vi "lia_host_chebyshev.vi"() -> ()   [LabVIEW 2009]
uses:
  <vilib>/rvi/interface/nirviOpenFPGA/nirviOpenFPGA.xnode
  FPGA Bitfiles/test_lia.lvproj_FPGA Target_lia_fpga_array.vi.lvbitx
  lia_fpga_array.vi
  <vilib>/FPGAPlugInAG/Pxi-7841r/nirviIntfOpen_PXI-7841R.vi
  <vilib>/rvi/interface/nirviMethod/nirviMethod.xnode
  <vilib>/Utility/error.llb/Merge Errors.vi
  <vilib>/LabVIEW Targets/FPGA/Rio/nirio_HostInterface/nirio_DMAStopAll.vi
  <vilib>/rvi/interface/common/niFpgaNodeNameForErrorReporting.ctl
  <vilib>/rvi/errors/niLvFpgaWhatHappensToTopLevelVI.ctl
  <vilib>/LabVIEW Targets/FPGA/Rio/nirio_HostInterface/nirio_DisableInterrupts.vi
  <vilib>/Utility/error.llb/Error Cluster From Error Code.vi
  <vilib>/rvi/errors/niLvFpgaAdjustHostInterfaceError.vi
  <vilib>/LabVIEW Targets/FPGA/Rio/nirio_HostInterface/nirio_Reset.vi
  <vilib>/RVI Host/nirviSupport.llb/nirviErrorClusterFromErrorCode.vi
  <vilib>/LabVIEW Targets/FPGA/Rio/nirio_HostInterface/nirio_EnableInterrupts.vi
  <vilib>/rvi/errors/niLvFpgaReportInternalErrorWithAdditionalInfo.vi
  <vilib>/rvi/interface/nirviReadWriteControl/nirviReadWriteControl.xnode
  <vilib>/LabVIEW Targets/FPGA/Rio/nirio_HostInterface/nirio_WriteBig.vi
  <vilib>/LabVIEW Targets/FPGA/Rio/nirio_HostInterface/nirio_ReadBig.vi
  <vilib>/rvi/interface/nirviCloseFPGA/nirviCloseFPGA.xnode
  <vilib>/FPGAPlugInAG/Pxi-7841r/nirviIntfClose_PXI-7841R.vi
  <vilib>/userDefined/High Color/nirio_resource_hc.ctl
  NiRioSrv.dll
panel:
  in  "Time Constant [s] 4":dbl caption="Time Constant [s]"
  out "Y [V] 4":dbl caption="Y [V]"
  out "Phase [Deg] 4":dbl caption="Phase [Deg]"
  out "R [V] 4":dbl caption="R [V]"
  out "X [V] 4":dbl
  in  "Filter Rolloff 4":enum8{"6 dB", "12 dB", "18 dB", "24 dB"}(ring) caption="Filter Rolloff"
  in  "Amplitude [V] 4":dbl caption="Amplitude [V]"
  in  "Frequency [Hz] 4":dbl caption="Frequency [Hz]"
  in  "Phase Shift [Deg] 4":dbl caption="Phase Shift [Deg]"
  in  "Time Constant [s] 3":dbl caption="Time Constant [s]"
  out "Y [V] 3":dbl caption="Y [V]"
  out "Phase [Deg] 3":dbl caption="Phase [Deg]"
  out "R [V] 3":dbl caption="R [V]"
  out "X [V] 3":dbl
  in  "Filter Rolloff 3":enum8{"6 dB", "12 dB", "18 dB", "24 dB"}(ring) caption="Filter Rolloff"
  in  "Amplitude [V] 3":dbl caption="Amplitude [V]"
  in  "Frequency [Hz] 3":dbl caption="Frequency [Hz]"
  in  "Phase Shift [Deg] 3":dbl caption="Phase Shift [Deg]"
  in  "Time Constant [s] 2":dbl caption="Time Constant [s]"
  out "Y [V] 2":dbl caption="Y [V]"
  out "Phase [Deg] 2":dbl caption="Phase [Deg]"
  out "R [V] 2":dbl caption="R [V]"
  out "X [V] 2":dbl
  in  "Filter Rolloff 2":enum8{"6 dB", "12 dB", "18 dB", "24 dB"}(ring) caption="Filter Rolloff"
  in  "Amplitude [V] 2":dbl caption="Amplitude [V]"
  in  "Frequency [Hz] 2":dbl caption="Frequency [Hz]"
  in  "Phase Shift [Deg] 2":dbl caption="Phase Shift [Deg]"
  in  "Time Constant [s]":dbl
  out "Y [V]":dbl
  out "Phase [Deg]":dbl
  out "R [V]":dbl
  out "X [V]":dbl
  in  "Data Rate [Hz]":dbl
  in  "Filter Rolloff":enum8{"6 dB", "12 dB", "18 dB", "24 dB"}(ring)
  in  "stop":bool
  in  "Update Freq [Hz]":dbl
  in  "Amplitude [V]":dbl
  in  "Frequency [Hz]":dbl
  in  "Phase Shift [Deg]":dbl
  # "Lockin Amplifier 1"
  # "Lockin Amplifier 3"
  # "Filter Settings"
  # "Output"
  # "Filter Settings"
  # "Output"
  # "Reference Signal Settings"
  # "Reference Signal Settings"
  # "Lockin Amplifier 2"
  # "Lockin Amplifier 4"
  # "Filter Settings"
  # "Output"
  # "Filter Settings"
  # "Output"
  # "Global"
  # "Reference Signal Settings"
  # "Reference Signal Settings"
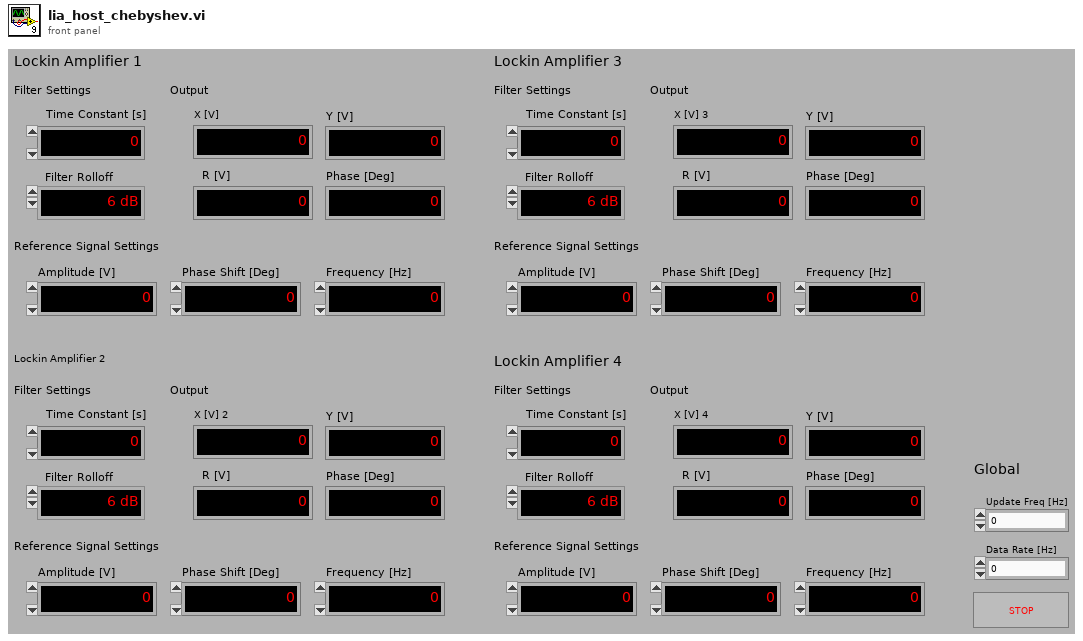
[diagram p1: front panel]
types:
  T1 = typedef "niFpgaNodeNameForErrorReporting.ctl" = enum16{"Open FPGA VI Reference", "Read/Write Control", "Invoke Method: Abort", "Invoke Method: Acknowledge IRQ", "Invoke Method: Download", "Invoke Method: FIFO.Configure", "Invoke Method: FIFO.Read", "Invoke Method: FIFO.Start", "Invoke Method: FIFO.Stop", "Invoke Method: FIFO.Write", "Invoke Method: Reset", "Invoke Method: Run", "Invoke Method: Wait on IRQ", "Close FPGA VI Reference"}
  T2 = typedef "niLvFpgaWhatHappensToTopLevelVI.ctl" = enum16{"top level VI scripted behind XNode", "top level VI inlined behind XNode"}
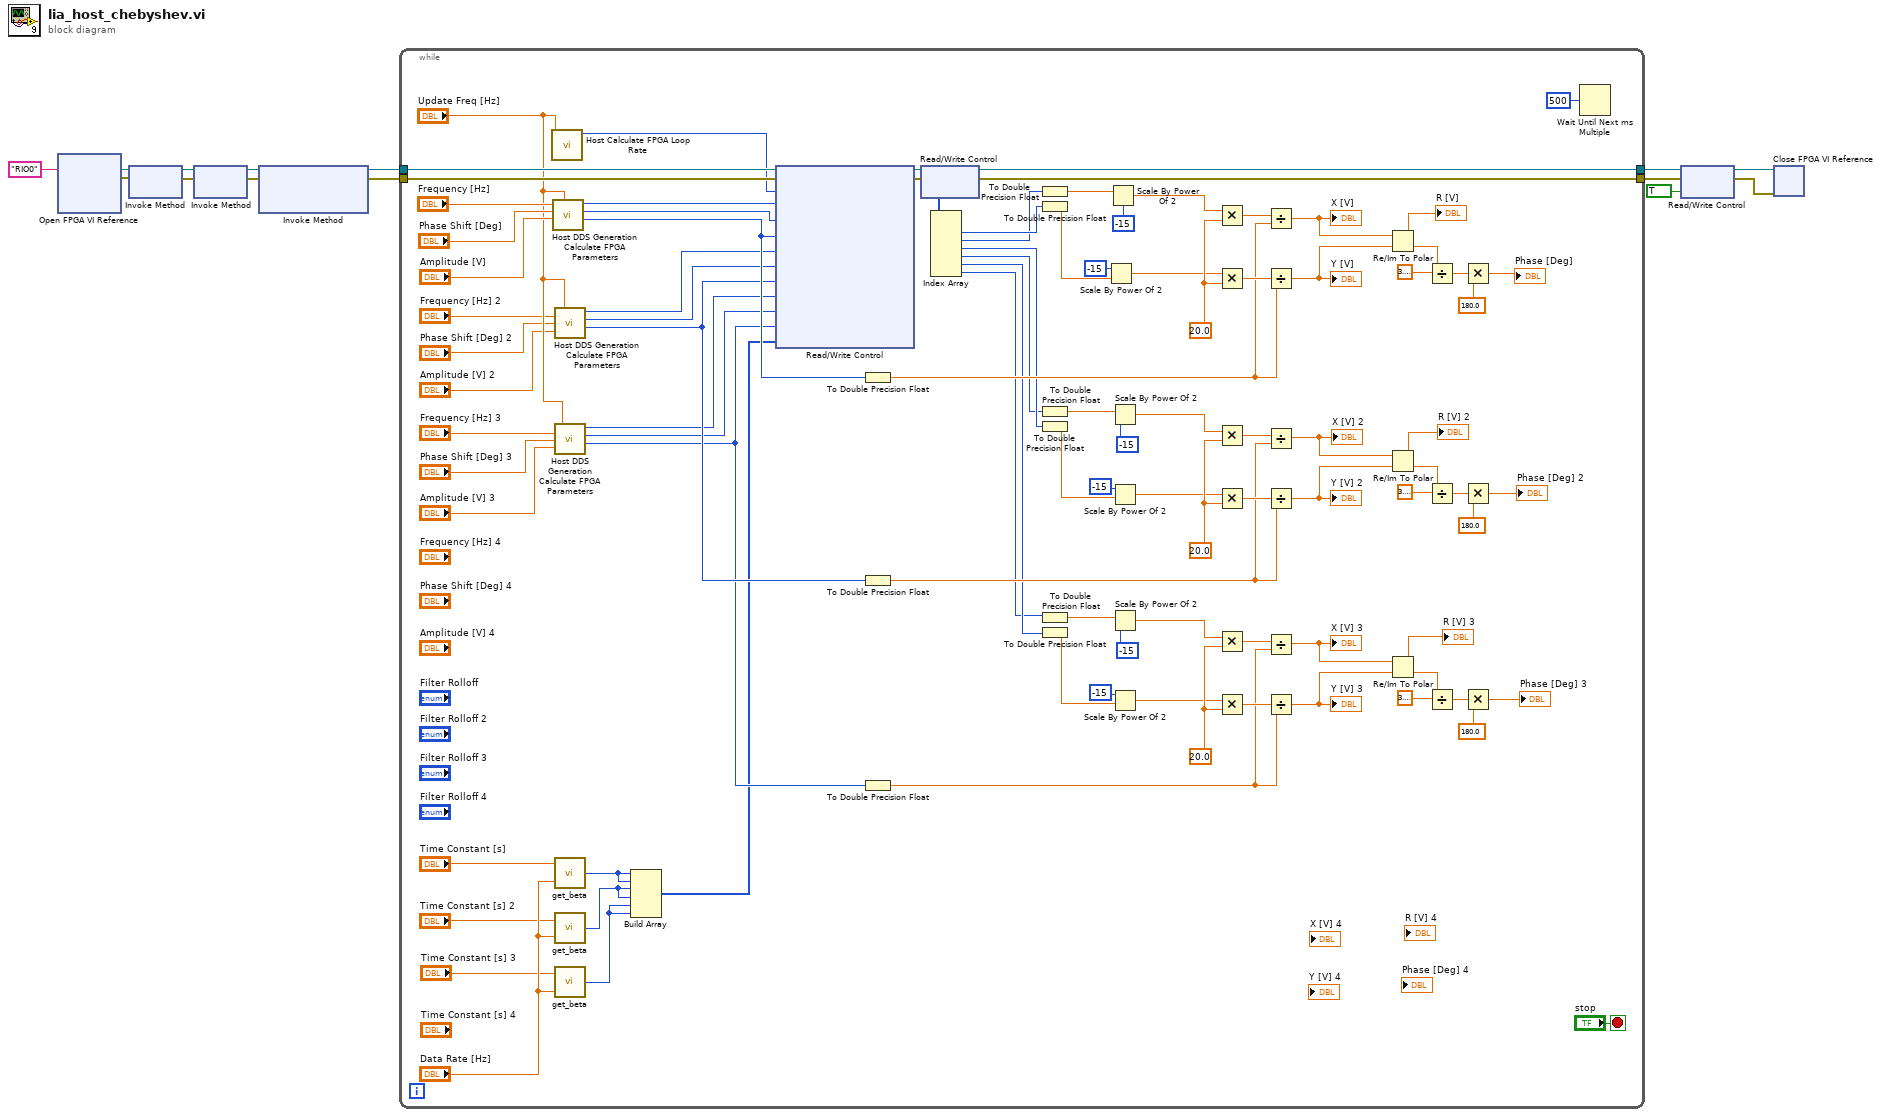
[diagram p0: block diagram]
diagram:
  n1 = xnode "Open FPGA VI Reference"("resource name"="RIO0") -> ("FPGA VI Reference Out"=w9:refnum<k20>, "error out"=w8:errorcluster)  [unwired: 1 in]
  n2 = xnode "Invoke Method"("FPGA VI Reference In"=w9, "error in"=w8) -> ("FPGA VI Reference Out"=w13:refnum<k20>, "error out"=w12:errorcluster)
  n3 = xnode "Invoke Method"("FPGA VI Reference In"=w13, "error in"=w12) -> ("FPGA VI Reference Out"=w11:refnum<k20>, "error out"=w10:errorcluster)
  n4 = xnode "Invoke Method"("FPGA VI Reference In"=w11, "error in"=w10) -> ("FPGA VI Reference Out"=w7:refnum<k20>, "error out"=w6:errorcluster)  [unwired: 1 out]
  n5 = while {
    tunnel: w7 -> [w107]
    tunnel: w6 -> [w106]
    tunnel: [w100] -> w3
    tunnel: [w99] -> w2
    stop <- "stop" stop-if-true
    w56 = 20.0
    w82 = 20.0
    w74 = 20.0
    n6 = call "Host Calculate FPGA Loop Rate.vi"("Loop Frequency (Hz)"="Update Freq [Hz]") -> ("Loop  Rate (ticks)"=w105:u32)  [unwired: 10 in]
    n7 = call "Host DDS Generation Calculate FPGA Parameters.vi"("Loop Rate (Hz)"="Update Freq [Hz]", "Signal Amplitude (V)"="Amplitude [V]", "Phase Shift (Deg)"="Phase Shift [Deg]", "DDS Signal Frequency (Hz)"="Frequency [Hz]") -> ("AO Amplitude"=w93:u16, "Phase Shift Sin"=w103:u32, "Accumulator Increment"=w104:u32)  [unwired: 3 in, 2 out]
    n8 = call "Host DDS Generation Calculate FPGA Parameters.vi"("Loop Rate (Hz)"="Update Freq [Hz]", "Signal Amplitude (V)"="Amplitude [V] 2", "Phase Shift (Deg)"="Phase Shift [Deg] 2", "DDS Signal Frequency (Hz)"="Frequency [Hz] 2") -> ("AO Amplitude"=w77:u16, "Phase Shift Sin"=w85:u32, "Accumulator Increment"=w86:u32)  [unwired: 3 in, 2 out]
    n9 = call "Host DDS Generation Calculate FPGA Parameters.vi"("Loop Rate (Hz)"="Update Freq [Hz]", "Signal Amplitude (V)"="Amplitude [V] 3", "Phase Shift (Deg)"="Phase Shift [Deg] 3", "DDS Signal Frequency (Hz)"="Frequency [Hz] 3") -> ("AO Amplitude"=w45:u16, "Phase Shift Sin"=w59:u32, "Accumulator Increment"=w60:u32)  [unwired: 3 in, 2 out]
    n10 = call "get_beta.vi"("Data Rate [Hz]"="Data Rate [Hz]", "Time Constant [s]"="Time Constant [s]") -> ("beta"=w43:i32)
    n11 = call "get_beta.vi"("Data Rate [Hz]"="Data Rate [Hz]", "Time Constant [s]"="Time Constant [s] 2") -> ("beta"=w42:i32)
    n12 = call "get_beta.vi"("Data Rate [Hz]"="Data Rate [Hz]", "Time Constant [s]"="Time Constant [s] 3") -> ("beta"=w41:i32)
    n13 = Build Array(w43, w43, w42, w42, w41, w41) -> (w40:i32[])
    n14 = xnode "Read/Write Control"("FPGA VI Reference In"=w107, "error in"=w106, "Update Rate (ticks)"=w105, "Accumulator Increment 1"=w104, "Phase Shift 1"=w103, "Signal Amplitude 1"=w93, "Accumulator Increment 2"=w86, "Phase Shift 2"=w85, "Signal Amplitude 2"=w77, "Accumulator Increment 3"=w60, "Phase Shift 3"=w59, "Signal Amplitude 3"=w45, "beta"=w40) -> ("FPGA VI Reference Out"=w102:refnum<k20>, "error out"=w101:errorcluster)
    n15 = To Double Precision Float(number=w93) -> (double precision float=w92:dbl)
    n16 = To Double Precision Float(number=w77) -> (double precision float=w76:dbl)
    n17 = To Double Precision Float(number=w45) -> (double precision float=w44:dbl)
    n18 = xnode "Read/Write Control"("FPGA VI Reference In"=w102, "error in"=w101) -> ("FPGA VI Reference Out"=w100:refnum<k20>, "error out"=w99:errorcluster, "XY_fpga"=w39:i32[])
    n19 = Index Array(array=w39) -> (element #1=w38:i32, element #2=w37:i32, element #3=w36:i32, element #4=w35:i32, element #5=w34:i32, element #6=w33:i32)  [unwired: 6 in]
    n20 = To Double Precision Float(number=w37) -> (double precision float=w70:dbl)
    n21 = To Double Precision Float(number=w38) -> (double precision float=w72:dbl)
    n22 = To Double Precision Float(number=w35) -> (double precision float=w67:dbl)
    n23 = To Double Precision Float(number=w36) -> (double precision float=w64:dbl)
    n24 = To Double Precision Float(number=w33) -> (double precision float=w51:dbl)
    n25 = To Double Precision Float(number=w34) -> (double precision float=w48:dbl)
    n26 = Scale By Power Of 2(n=-15, x=w72) -> (x*2^n=w73:dbl)
    n27 = Scale By Power Of 2(n=-15, x=w70) -> (x*2^n=w68:dbl)
    n28 = Scale By Power Of 2(n=-15, x=w67) -> (x*2^n=w66:dbl)
    n29 = Scale By Power Of 2(n=-15, x=w64) -> (x*2^n=w63:dbl)
    n30 = Scale By Power Of 2(n=-15, x=w51) -> (x*2^n=w50:dbl)
    n31 = Scale By Power Of 2(n=-15, x=w48) -> (x*2^n=w47:dbl)
    n32 = Multiply(x=w68, y=w74) -> (x*y=w98:dbl)
    n33 = Multiply(x=w73, y=w74) -> (x*y=w97:dbl)
    n34 = Multiply(x=w66, y=w82) -> (x*y=w84:dbl)
    n35 = Multiply(x=w63, y=w82) -> (x*y=w83:dbl)
    n36 = Multiply(x=w50, y=w56) -> (x*y=w58:dbl)
    n37 = Multiply(x=w47, y=w56) -> (x*y=w57:dbl)
    n38 = Divide(x=w98, y=w92) -> (x/y=w96:dbl)
    "X [V]" <- w96
    n39 = Divide(x=w97, y=w92) -> (x/y=w95:dbl)
    "Y [V]" <- w95
    n40 = Divide(x=w84, y=w76) -> (x/y=w15:dbl)
    "X [V] 2" <- w15
    n41 = Divide(x=w83, y=w76) -> (x/y=w16:dbl)
    "Y [V] 2" <- w16
    n42 = Divide(x=w58, y=w44) -> (x/y=w22:dbl)
    "X [V] 3" <- w22
    n43 = Divide(x=w57, y=w44) -> (x/y=w21:dbl)
    "Y [V] 3" <- w21
    n44 = Re/Im To Polar(2:w95, 3:w96) -> (0:w91:dbl, 1:→"R [V]":dbl)
    n45 = Re/Im To Polar(2:w16, 3:w15) -> (0:w81:dbl, 1:→"R [V] 2":dbl)
    n46 = Re/Im To Polar(2:w21, 3:w22) -> (0:w55:dbl, 1:→"R [V] 3":dbl)
    n47 = Divide(x=w91, y=3.141592653589793) -> (x/y=w89:dbl)
    n48 = Divide(x=w81, y=3.141592653589793) -> (x/y=w79:dbl)
    n49 = Divide(x=w55, y=3.141592653589793) -> (x/y=w53:dbl)
    n50 = Multiply(x=w89, y=180.0) -> (x*y=→"Phase [Deg]":dbl)
    n51 = Multiply(x=w79, y=180.0) -> (x*y=→"Phase [Deg] 2":dbl)
    n52 = Multiply(x=w53, y=180.0) -> (x*y=→"Phase [Deg] 3":dbl)
    n53 = Wait Until Next ms Multiple(millisecond multiple=u32 500) -> ()  [unwired: 1 out]
  }
  n54 = xnode "Read/Write Control"("FPGA VI Reference In"=w3, "error in"=w2, "stop"=TRUE) -> ("FPGA VI Reference Out"=w5:refnum<k20>, "error out"=w4:errorcluster)
  n55 = xnode "Close FPGA VI Reference"("FPGA VI Reference In"=w5, "error in"=w4) -> ()  [unwired: 1 out]
